vi "command_encoder.vi"(0 "String in":string, 1 "Numeric":i32, 2 "Speed":dbl, 3 "Numeric 2":i32) -> (7 "String out":string)   [LabVIEW 2017]
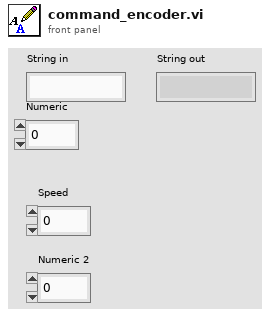
[diagram p1: front panel]
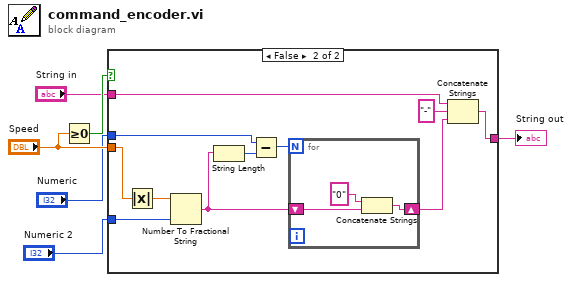
[diagram p0: block diagram]
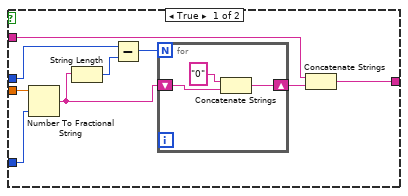
[diagram p2: hidden frame]
diagram:
  n1 = Greater Or Equal To 0?(x="Speed") -> (x >= 0?=w6:bool)
  n2 = case shown="False" w6 {
    tunnel: "Speed" -> [w11 w21]
    tunnel: [w10 w26] -> w4
    tunnel: "Numeric" -> [w9 w25]
    tunnel: "Numeric 2" -> [w8 w24]
    tunnel: "String in" -> [w7 w23]
    frame True {
      n3 = Number To Fractional String(number=w11, precision (6)=w8) -> (F-format string=w13:string)  [unwired: 2 in]
      n4 = String Length(string=w13) -> (length=w15:i32)
      n5 = Subtract(x=w9, y=w15) -> (x-y=w14:i32)
      n6 = for {
        N: w14 -> [_]
        shift-right: [w16] -> w12
        shift-left: w13 -> [w17]
        n7 = Concatenate Strings("0", w17) -> (w16:string)
      }
      n8 = Concatenate Strings(w7, w12) -> (w10:string)
    }
    frame False {
      n9 = Absolute Value(x=w21) -> (abs(x)=w22:dbl)
      n10 = Number To Fractional String(number=w22, precision (6)=w24) -> (F-format string=w27:string)  [unwired: 2 in]
      n11 = String Length(string=w27) -> (length=w29:i32)
      n12 = Subtract(x=w25, y=w29) -> (x-y=w28:i32)
      n13 = for {
        N: w28 -> [_]
        shift-right: [w30] -> w20
        shift-left: w27 -> [w31]
        n14 = Concatenate Strings("0", w31) -> (w30:string)
      }
      n15 = Concatenate Strings(w23, "-", w20) -> (w26:string)
    }
  }
  "String out" <- w4
